vi "Data to Single Line String.vi"(8 "error in (no error)":errorcluster, 11 "Report Data in":refnum<class "Report Data.lvclass">) -> (0 "error out":errorcluster, 3 "Single Line Data":string)   [LabVIEW 2020, in "ProjectBuilder.lvlib" / "Report Data.lvclass"]
uses:
  Report Data.lvclass
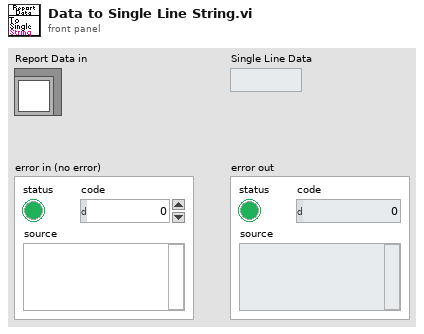
[diagram p1: front panel]
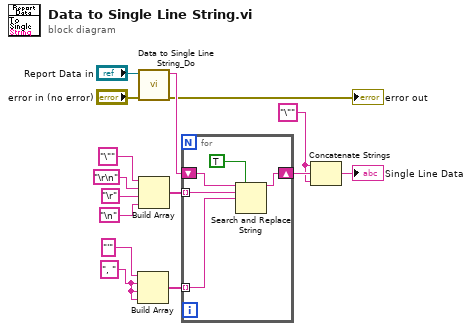
[diagram p0: block diagram]
diagram:
  w5 = ", " ("search string")
  w13 = "\"" ("search string")
  n1 = Build Array("'" ("search string"), w5, w5, w5) -> (w9:string[])
  n2 = call-dynamic "Data to Single Line String_Do.vi"("error in (no error)"="error in (no error)", "Report Data in"="Report Data in") -> ("error out"=→"error out":errorcluster, "String Data"=w3:string)  [unwired: 8 in]
  n3 = Build Array("\"" ("search string"), "\r\n", "\r", "\n") -> (w10:string[])
  n4 = for {
    tunnel: w9 -> [w18] mode=indexing
    tunnel: w10 -> [w17] mode=indexing
    shift-right: [w19] -> w15
    shift-left: w3 -> [w16]
    n5 = Search and Replace String(replace all?=TRUE ("replace all? (F)"), input string=w16, search string=w17, replace string=w18) -> (result string=w19:string)  [unwired: 4 in, 3 out]
  }
  n6 = Concatenate Strings(w13, w15, w13) -> (→"Single Line Data":string)
